vi "Delete Int32 DVR.vi"(8 "error in (no error)":errorcluster, 11 "Int32 DVR in":refnum<data-value>) -> (0 "error out":errorcluster, 3 "Int32 out":refnum<class " Int32.lvclass">)   [LabVIEW 2010, in "MDSplus.lvlib" / " Int32.lvclass"]
uses:
  <vilib>/MDSplus/Classes/Data_Class/Scalar_Class/Int32_Class/ Int32.lvclass
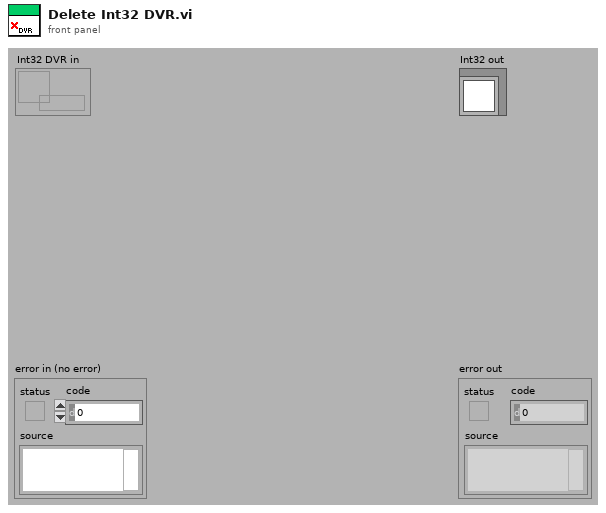
[diagram p1: front panel]
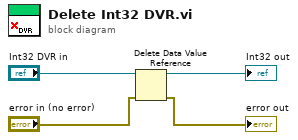
[diagram p0: block diagram]
diagram:
  n1 = Delete Data Value Reference(data value reference="Int32 DVR in", error in="error in (no error)") -> (data value=→"Int32 out":refnum<class " Int32.lvclass">, error out=→"error out":errorcluster)
